vi "getRoutings.vi"(8 "error in (no error)":errorcluster, 11 "DoDeviceData in":refnum<class "DoDeviceData.lvclass">) -> (0 "error out":errorcluster, 2 "Routings":cluster{"Master Clock Route":string[]}, 3 "DoDeviceData out":refnum<class "DoDeviceData.lvclass">)   [LabVIEW 2009, in "DataMappers.lvlib" / "DoDeviceData.lvclass"]
uses:
  DoDeviceData.lvclass
  DatabaseHelpers/Database Objects/device/DigitalDevice/DigitalDevice.lvclass
  DeviceData.lvclass
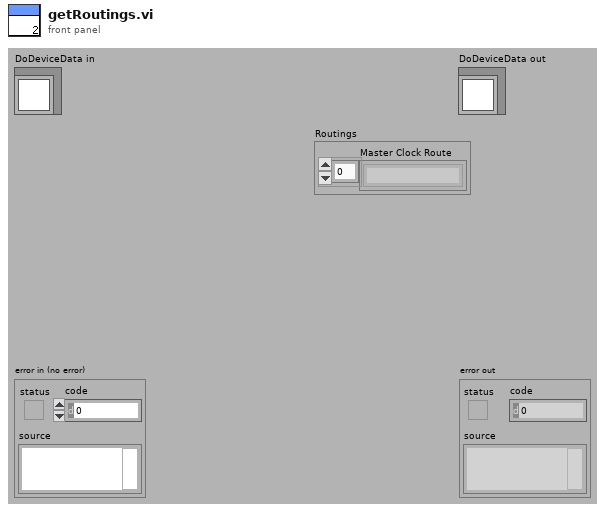
[diagram p1: front panel]
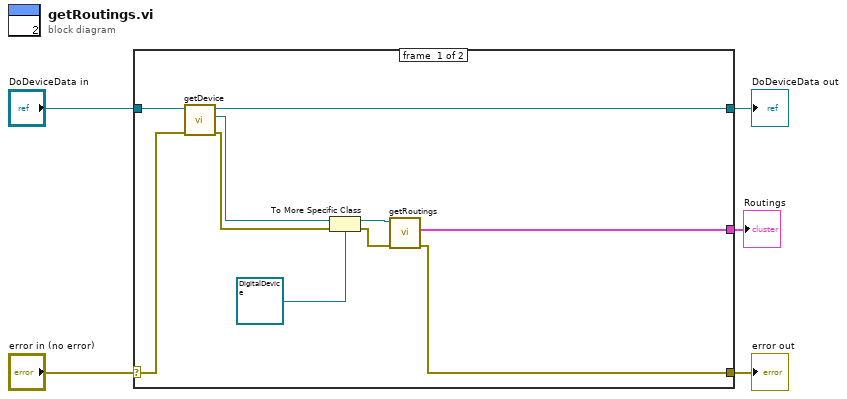
[diagram p0: block diagram]
diagram:
  n1 = case shown="No Error" "error in (no error)" {
    selector: "error in (no error)" -> [w8 w17]
    tunnel: [w6 w17] -> w4
    tunnel: [w14 w16] -> w2
    tunnel: "DoDeviceData in" -> [w15 w16]
    tunnel: [w7 _] -> w1
    frame #0 {
      n2 = call "getDevice.vi"("error in (no error)"=w8, "DeviceData.lvclass in"=w15) -> ("error out"=w9:errorcluster, "device"=w10:refnum<class "device.lvclass">, "DeviceData.lvclass out"=w14:refnum<class "DoDeviceData.lvclass">)  [unwired: 7 in]
      n3 = To More Specific Class(target class=refnum<class "DigitalDevice.lvclass"> refnum ("Tools.lvlib:DatabaseHelpers.lvlib:DigitalDevice.lvclass"), reference=w10, error in=w9) -> (specific class reference=w13:refnum<class "DigitalDevice.lvclass">, error out=w12:errorcluster)
      n4 = call "getRoutings.vi"("error in (no error)"=w12, "DigitalDevice.lvclass in"=w13) -> ("error out"=w6:errorcluster, "Routings"=w7:cluster{"Master Clock Route":string[]})  [unwired: 7 in, 1 out]
    }
    frame #1 {
    }
  }
  "error out" <- w4
  "DoDeviceData out" <- w2
  "Routings" <- w1
